vi "initboard.vi"(8 "error in (no error)":errorcluster, 10 "address":string="172.16.7.43", 11 "remote port or service name":u16=9764) -> (0 "error out":errorcluster)   [LabVIEW 2009]
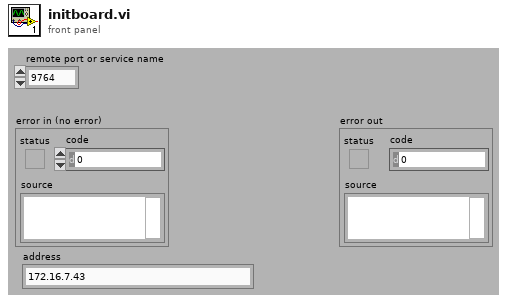
[diagram p1: front panel]
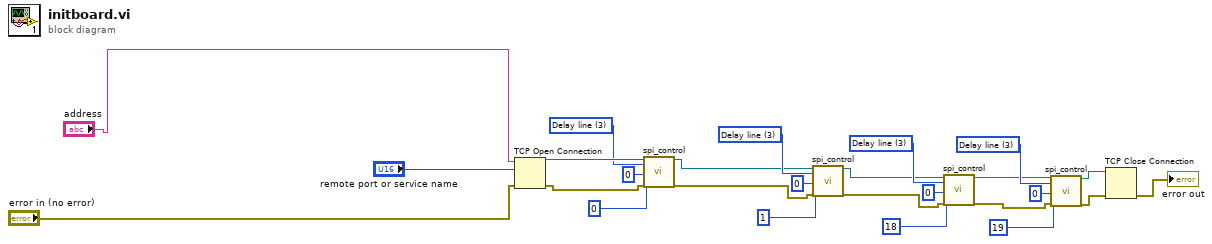
[diagram p0: block diagram]
diagram:
  w11 = u16 3 items=["Attenuation", "Clipping", "Enable channel", "Delay line", "ASIC"] ("Device")
  w14 = u16 3 items=["Attenuation", "Clipping", "Enable channel", "Delay line", "ASIC"] ("Device")
  w17 = u16 3 items=["Attenuation", "Clipping", "Enable channel", "Delay line", "ASIC"] ("Device")
  w20 = u16 3 items=["Attenuation", "Clipping", "Enable channel", "Delay line", "ASIC"] ("Device")
  n1 = TCP Open Connection(address="address", remote port or service name="remote port or service name", error in (no error)="error in (no error)") -> (connection ID=w21:refnum<k5>, error out=w22:errorcluster)  [unwired: 2 in]
  n2 = call "spi_control.vi"("connection ID"=w21, "Device"=w20, "Data"=0, "Register or channel"=0, "error out 3"=w22) -> ("connection ID out"=w8:refnum<k5>, "error out 2"=w7:errorcluster)  [unwired: 7 in, 6 out]
  n3 = call "spi_control.vi"("connection ID"=w8, "Device"=w17, "Data"=0, "Register or channel"=1, "error out 3"=w7) -> ("connection ID out"=w6:refnum<k5>, "error out 2"=w5:errorcluster)  [unwired: 7 in, 6 out]
  n4 = call "spi_control.vi"("connection ID"=w6, "Device"=w14, "Data"=0, "Register or channel"=18, "error out 3"=w5) -> ("connection ID out"=w4:refnum<k5>, "error out 2"=w3:errorcluster)  [unwired: 7 in, 6 out]
  n5 = call "spi_control.vi"("connection ID"=w4, "Device"=w11, "Data"=0, "Register or channel"=19, "error out 3"=w3) -> ("connection ID out"=w1:refnum<k5>, "error out 2"=w2:errorcluster)  [unwired: 7 in, 6 out]
  n6 = TCP Close Connection(connection ID=w1, error in (no error)=w2) -> (error out=→"error out":errorcluster)  [unwired: 1 in, 1 out]
